vi "Part 1.vi"(11 "Input":string) -> (3 "Output":i64)   [LabVIEW 2021]
uses:
  <userlib>/_OpenG.lib/string/string.llb/Convert EOLs (String)__ogtk.vi
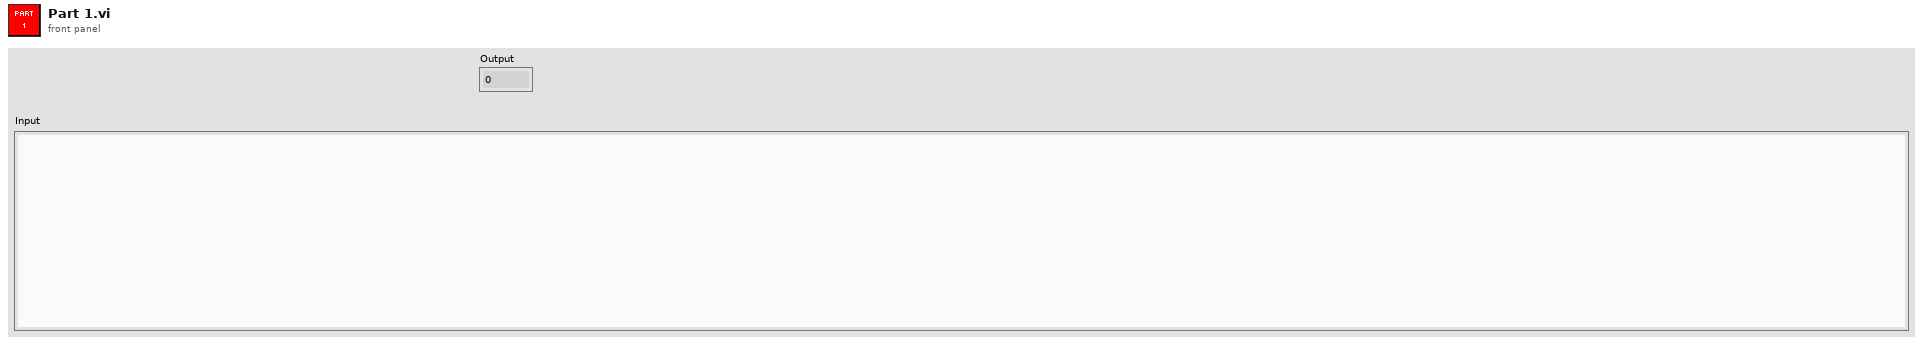
[diagram p1: front panel]
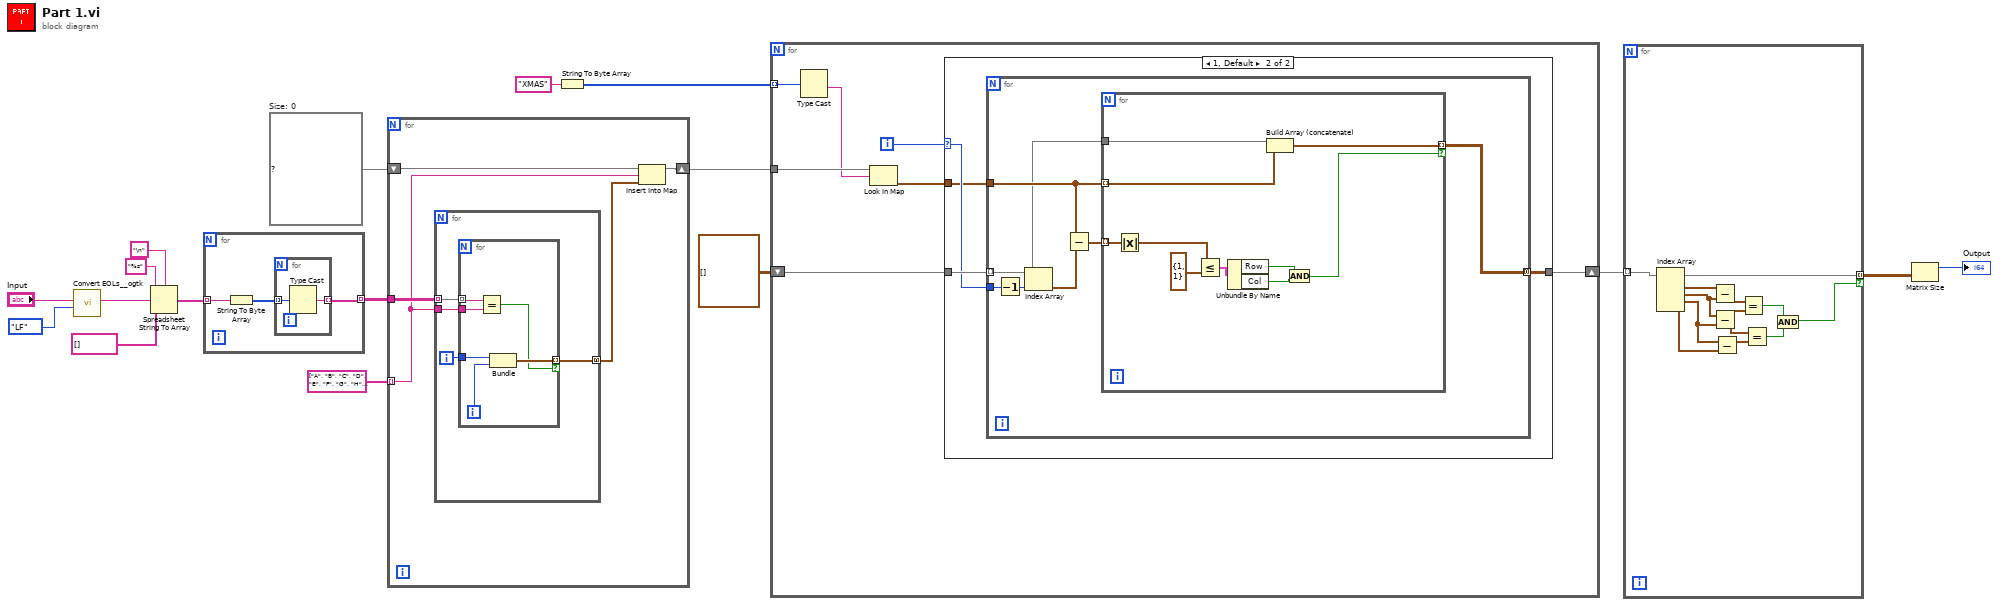
[diagram p0: block diagram]
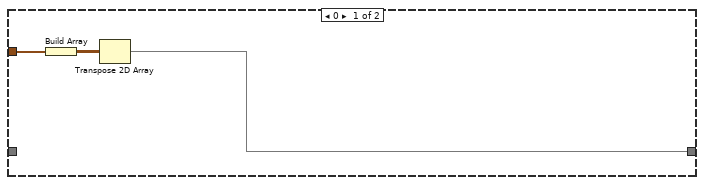
[diagram p2: hidden frame]
diagram:
  w8 = map{string, cluster{"Row":i32, "Col":i32}[]} {}  # Size: 0
  n1 = call-poly <userlib>:"Convert EOLs__ogtk.vi"("Convert to:"=enum16{"CR", "LF", "CRLF"}."LF", "String in"="Input") -> ("String out"=w13:string)  [unwired: 9 in]
  n2 = Spreadsheet String To Array(delimiter (Tab)="\n", format string="%s", spreadsheet string=w13, array type (2D Dbl)=string[] []) -> (array=w11:string[])
  n3 = for {
    tunnel: w11 -> [w20] mode=indexing
    tunnel: [w18] -> w10 mode=indexing
    n4 = String To Byte Array(string=w20) -> (unsigned byte array=w19:u8[])
    n5 = for {
      tunnel: w19 -> [w22] mode=indexing
      tunnel: [w21] -> w18 mode=indexing
      n6 = Type Cast(x=w22) -> (*(type *) &x=w21:string)  [unwired: 1 in]
    }
  }
  n7 = for {
    tunnel: w10 -> [w25]
    tunnel: string[] ["A", "B", "C", "D", "E", "F", "G", "H", "I", "J", "K", "L", "M", "N", "O", "P", "Q", "R", "S", "T", "U", "V", "W", "X", "Y", "Z"] ("Array") -> [w24] mode=indexing
    shift-right: [w27] -> w7
    shift-left: w8 -> [w26]
    n8 = for {
      tunnel: w25 -> [w31] mode=indexing
      tunnel: w24 -> [w30]
      tunnel: [w28] -> w23 mode=concatenating
      i -> [w29]
      n9 = for {
        tunnel: w31 -> [w37] mode=indexing
        tunnel: w30 -> [w36]
        tunnel: w29 -> [w35]
        tunnel: [w33] -> w28 mode=indexing if=w32
        i -> [w34]
        n10 = Equal?(x=w37, y=w36) -> (x = y?=w32:bool)
        n11 = Bundle(w35, w34) -> (w33:cluster{i32, i32})  [unwired: 1 in]
      }
    }
    n12 = Insert Into Map(map in=w26, key=w24, value=w23) -> (map out=w27:map{string, cluster{"Row":i32, "Col":i32}[]})  [unwired: 2 out]
  }
  n13 = String To Byte Array(string="XMAS") -> (unsigned byte array=w5:u8[])
  n14 = for {
    tunnel: w7 -> [w43]
    tunnel: w5 -> [w44] mode=indexing
    shift-right: [w39] -> w2
    shift-left: cluster{"Row":i32, "Col":i32}[][] [] -> [w38]
    i -> [w40]
    n15 = Type Cast(x=w44) -> (*(type *) &x=w42:string)  [unwired: 1 in]
    n16 = Look In Map(map=w43, key=w42) -> (value=w41:cluster{"Row":i32, "Col":i32}[])  [unwired: 1 in, 1 out]
    n17 = case shown="1, Default" w40 {
      selector: w40 -> [_ w50]
      tunnel: w41 -> [w47 w49]
      tunnel: [w45 w48] -> w39
      tunnel: w38 -> [_ w51]
      frame 0 {
        n18 = Build Array(w47) -> (w46:cluster{"Row":i32, "Col":i32}[][])
        n19 = Transpose 2D Array(2D array=w46) -> (transposed array=w45:cluster{"Row":i32, "Col":i32}[][])
      }
      frame 1, Default {
        n20 = for {
          tunnel: w51 -> [w53] mode=indexing
          tunnel: w50 -> [w58]
          tunnel: w49 -> [w54]
          tunnel: [w52] -> w48 mode=concatenating
          n21 = Decrement(x=w58) -> (x-1=w57:i32)
          n22 = Index Array(array=w53, index=w57) -> (element=w56:cluster{"Row":i32, "Col":i32})
          n23 = Subtract(x=w54, y=w56) -> (x-y=w55:cluster{"Row":i32, "Col":i32}[])
          n24 = for {
            tunnel: w55 -> [w67] mode=indexing
            tunnel: w54 -> [w66] mode=indexing
            tunnel: w53 -> [w68]
            tunnel: [w65] -> w52 mode=indexing if=w59
            n25 = Absolute Value(x=w67) -> (abs(x)=w64:cluster{"Row":i32, "Col":i32})
            n26 = Less Or Equal?(x=w64, y=cluster{"Row":i32, "Col":i32} {"Row"=1, "Col"=1}) -> (x <= y?=w62:cluster{"Row":bool, "Col":bool})
            n27 = Unbundle By Name(w62) -> ("Row"=w61:bool, "Col"=w60:bool)
            n28 = Build Array (concatenate)(w68, w66) -> (w65:cluster{"Row":i32, "Col":i32}[])
            n29 = And(x=w61, y=w60) -> (x .and. y?=w59:bool)
          }
        }
      }
    }
  }
  n30 = for {
    tunnel: w2 -> [w70] mode=indexing
    tunnel: [w70] -> w1 mode=indexing if=w69
    n31 = Index Array(array=w70) -> (element #1=w79:cluster{"Row":i32, "Col":i32}, element #2=w78:cluster{"Row":i32, "Col":i32}, element #3=w77:cluster{"Row":i32, "Col":i32}, element #4=w76:cluster{"Row":i32, "Col":i32})  [unwired: 4 in]
    n32 = Subtract(x=w79, y=w78) -> (x-y=w75:cluster{"Row":i32, "Col":i32})
    n33 = Subtract(x=w78, y=w77) -> (x-y=w73:cluster{"Row":i32, "Col":i32})
    n34 = Subtract(x=w77, y=w76) -> (x-y=w74:cluster{"Row":i32, "Col":i32})
    n35 = Equal?(x=w75, y=w73) -> (x = y?=w71:bool)
    n36 = Equal?(x=w73, y=w74) -> (x = y?=w72:bool)
    n37 = And(x=w71, y=w72) -> (x .and. y?=w69:bool)
  }
  n38 = Matrix Size(0:w1) -> (1:→"Output":i32)  [unwired: 1 out]
